vi "Assert Register Panel.vi"() -> ()   [LabVIEW 2015, in "Login.lvclass"]
uses:
  Login.lvclass
  API/_Database/Database.lvclass
  <vilib>/addons/database/Auxilliary.llb/DB Tools Column Info.ctl
  <vilib>/addons/database/Auxilliary.llb/DB Tools DataTypes.ctl
  Login.lvclass/Login.ctl
  <vilib>/addons/database/NI_Database_API.lvlib
panel:
  in  "Login in":refnum<class "Login.lvclass">
  in  "path":path=path "E:/哈工大竞技机器人队/机器人队管理系统/Database/CRTDatabase.accdb"
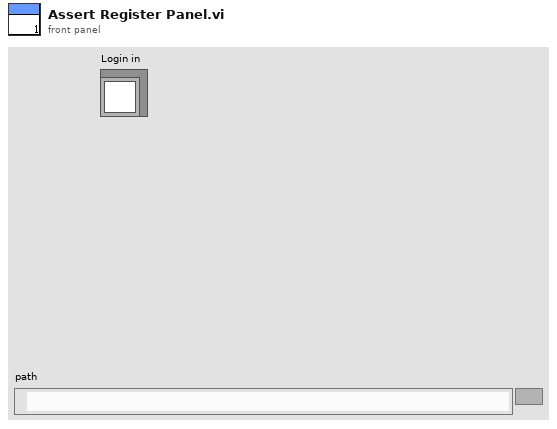
[diagram p1: front panel]
types:
  T1 = typedef "NI_Database_API.lvlib/DB Tools Column Info.ctl" = cluster{"column name":string, "data type":T2, "size":i32, "allow null?":bool}
  T2 = typedef "NI_Database_API.lvlib/DB Tools DataTypes.ctl" = enum16{"String", "Long (I32)", "Single (SGL)", "Double (DBL)", "Date/Time", "Binary"}
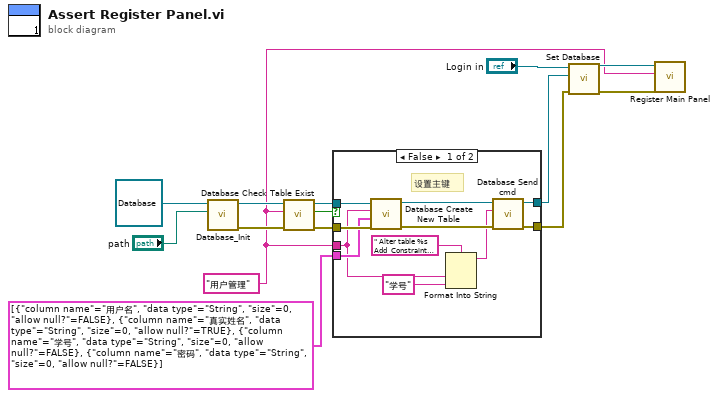
[diagram p0: block diagram]
diagram:
  w1 = "用户管理" ("Table")
  n1 = call "Database_Init.vi"("path"="path", "object in"=refnum<class "Database.lvclass"> refnum ("Database")) -> ("error out"=w11:errorcluster, "object out"=w12:refnum<class "Database.lvclass">)  [unwired: 8 in]
  n2 = call "Database Check Table Exist.vi"("error in (no error)"=w11, "Table"=w1, "Database in"=w12) -> ("error out"=w8:errorcluster, "Exit?"=w10:bool, "Database out"=w9:refnum<class "Database.lvclass">)  [unwired: 6 in]
  n3 = case shown="False" w10 {
    tunnel: w9 -> [w25 w27]
    tunnel: w8 -> [w24 w26]
    tunnel: w1 -> [w18 _]
    tunnel: T1[] [{"column name"="用户名", "data type"=enum."String", "size"=0, "allow null?"=FALSE}, {"column name"="真实姓名", "data type"=enum."String", "size"=0, "allow null?"=TRUE}, {"column name"="学号", "data type"=enum."String", "size"=0, "allow null?"=FALSE}, {"column name"="密码", "data type"=enum."String", "size"=0, "allow null?"=FALSE}] ("column information") -> [w23 _]
    tunnel: [w16 w26] -> w5
    tunnel: [w15 w27] -> w6
    frame False {
      # "设置主键"
      n4 = call "Database Create New Table.vi"("error in (no error)"=w24, "column information"=w23, "table"=w18, "Database in"=w25) -> ("error out"=w21:errorcluster, "Database out"=w22:refnum<class "Database.lvclass">)  [unwired: 6 in]
      n5 = Format Into String(format string=" Alter table %s Add  Constraint  PrimaryKey  Primary  Key (%s)" ("SQL query"), w18, "学号" ("input 2")) -> (resulting string=w17:string)  [unwired: 2 in, 1 out]
      n6 = call "Database Send cmd.vi"("error in (no error)"=w21, "SQL query"=w17, "Database in"=w22) -> ("error out"=w16:errorcluster, "Database out"=w15:refnum<class "Database.lvclass">)  [unwired: 7 in]
    }
    frame True {
    }
  }
  n7 = call "Set Database.vi"("error in (no error)"=w5, "Database"=w6, "Login in"="Login in") -> ("error out"=w2:errorcluster, "Login out"=w3:refnum<class "Login.lvclass">)  [unwired: 7 in]
  n8 = call "Register Main Panel.vi"("error in (no error)"=w2, "TableName"=w1, "Login.lvclass"=w3) -> ()  [unwired: 7 in, 2 out]
